vi "Kinect Joystick to Distance.vi"(1 "Input":i8) -> (0 "Output":dbl=2.4901960784313726)   [LabVIEW 2011]
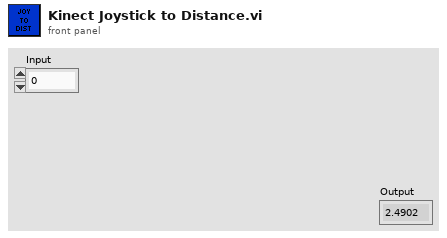
[diagram p1: front panel]
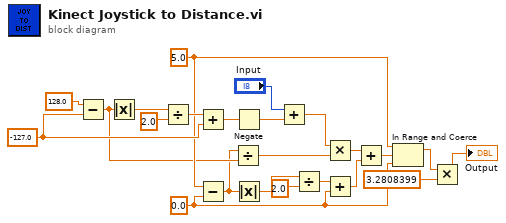
[diagram p0: block diagram]
diagram:
  w8 = 0.0 ("Output Min")
  w7 = 5.0 ("Output Max")
  w17 = -127.0 ("Input Min")
  n1 = Subtract(x=128.0 ("Input Max"), y=w17) -> (x-y=w5:dbl)
  n2 = Absolute Value(x=w5) -> (abs(x)=w23:dbl)
  n3 = Divide(x=w23, y=2.0 ("x")) -> (x/y=w18:dbl)
  n4 = Add(x=w18, y=w17) -> (x+y=w16:dbl)
  n5 = Subtract(x=w7, y=w8) -> (x-y=w4:dbl)
  n6 = Divide(x=w4, y=w5) -> (x/y=w12:dbl)
  n7 = Negate(x=w16) -> (-x=w20:dbl)
  n8 = Absolute Value(x=w4) -> (abs(x)=w22:dbl)
  n9 = Add(x="Input", y=w20) -> (x+y=w13:dbl)
  n10 = Divide(x=w22, y=2.0 ("x")) -> (x/y=w14:dbl)
  n11 = Multiply(x=w13, y=w12) -> (x*y=w11:dbl)
  n12 = Add(x=w14, y=w8) -> (x+y=w10:dbl)
  n13 = Add(x=w11, y=w10) -> (x+y=w9:dbl)
  n14 = In Range and Coerce(upper limit=w7, x=w9, lower limit=w8) -> (coerced(x)=w3:dbl)  [unwired: 1 out]
  n15 = Multiply(x=w3, y=3.2808399) -> (x*y=→"Output":dbl)
